vi "Connect.vi"(8 "error in (no error)":errorcluster, 11 "Ultimus V in":refnum<class "Ultimus V2.lvclass">) -> (0 "error out":errorcluster, 3 "Ultimus V out":refnum<class "Ultimus V2.lvclass">)   [LabVIEW 2016, in "Ultimus V2.lvclass"]
uses:
  Ultimus V2.lvclass
  Ultimus V2.lvclass/Ultimus V2.ctl
  Drivers/EFD Ultimus V/EFD Ultimus V.lvlib
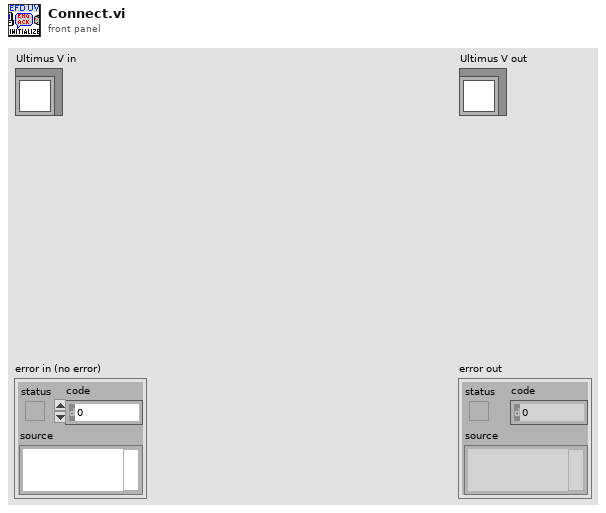
[diagram p1: front panel]
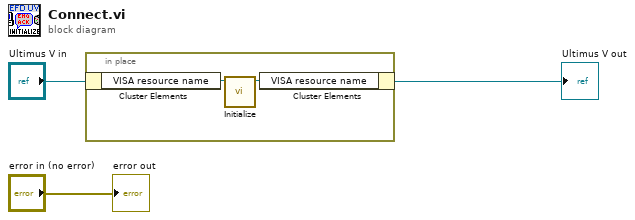
[diagram p0: block diagram]
diagram:
  n1 = in-place {
    n2 = in-place-cluster #1("Ultimus V in") -> ("VISA resource name"=w5:refnum<visa-resource-name>)
    n3 = call "Initialize.vi"("VISA resource name"=w5) -> ("VISA resource name out"=w4:refnum<visa-resource-name>)  [unwired: 9 in, 1 out]
    n4 = in-place-cluster #1("VISA resource name"=w4) -> (→"Ultimus V out":refnum<class "Ultimus V2.lvclass">)
  }
  "error out" <- "error in (no error)"
